vi "Keithley 6514 Digital Output Controls.vi"(0 "Resource In":refnum<visa-resource-name>, 1 "Check For SCPI Errors? (T)":bool=TRUE, 5 "Digital Output Control (Set Output Pattern:0)":u16(ring) items=["Set Output Pattern", "Clear Port Immediately", "Enable Auto-Clear Port", "Disable Auto-Clear Port", "Set Line-4 Mode Configuration"], 7 "4-Bit Digital\nOutput Pattern (1111b)":i8=15 min=0 max=15 step=1 format="%04b", 9 "Delay Pulse-Width for \nPass/Fail Pattern (0.0001 secs)":sgl=0.0001 min=0 max=60 step=0.0001 format="%.4f", 11 "error in (no error)":T1, 13 "Line 4 Mode (End of Test:T)":bool=TRUE, 14 "TTL Level for Busy (0:F)":bool) -> (4 "Resource Out":refnum<visa-resource-name>, 15 "error out":T1)   [LabVIEW 2009, in "Keithley 6514 LV 2009.lvlib"]
doc: "This VI is used to control the 4 digital output lines of the instrument. \n\nDigital Output Control:\n0 = Set Output Pattern\n1 = Clear Port Immediately\n2 = Enable Auto-Clear Port\n3 = Disable Auto-Clear Port\n4 = Set Line 4 Mode Configuration\n\n4-Bit Digital Output Pattern:\n0 to 15\n\nDelay Pulse-Width for Pass/Fail Pattern:\n0 to 60 (0.0001 Resolution)\n\nLine 4 Mode:\nTRUE = End of Test (EOT)'\nFALSE = Busy\n\nTTL Level for Busy:\nTRUE = 1 (HI)\nFALSE = 0 (LO)"
uses:
  Keithley 6514 LV 2009.lvlib
panel:
  # "End of Test\nBusy"
  # "1\n0"
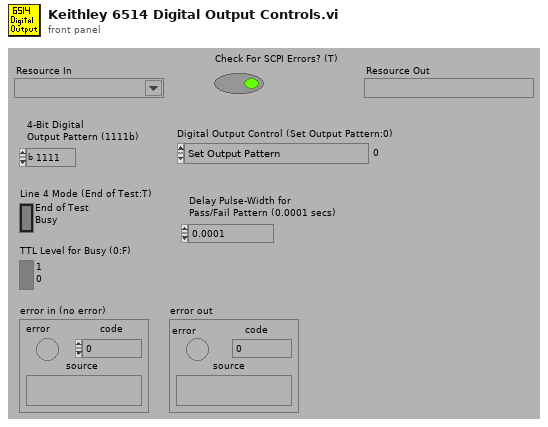
[diagram p1: front panel]
types:
  T1 = cluster{"error":bool, "code":i32, "source":string}
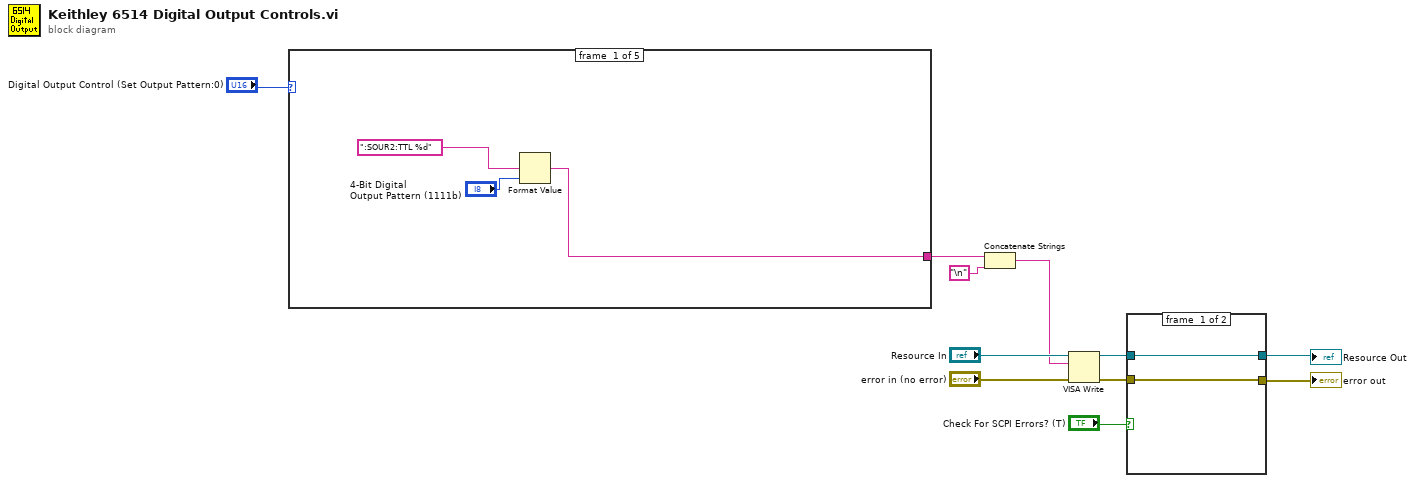
[diagram p0: block diagram]
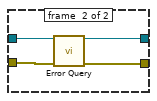
[diagram p2: hidden frame]
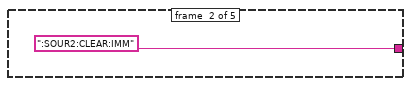
[diagram p3: hidden frame]
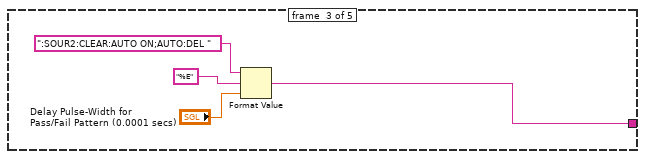
[diagram p4: hidden frame]
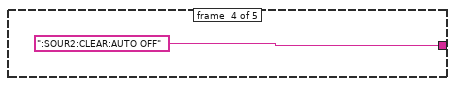
[diagram p5: hidden frame]
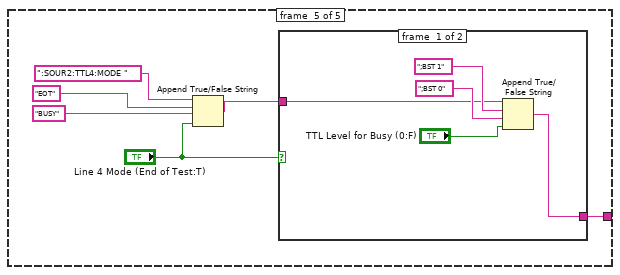
[diagram p6: hidden frame]
diagram:
  n1 = case shown="4" "Digital Output Control (Set Output Pattern:0)" {
    tunnel: [w12 ":SOUR2:CLEAR:IMM" w16 ":SOUR2:CLEAR:AUTO OFF" w21] -> w2
    frame #0 {
      n2 = Format Value(format string=":SOUR2:TTL %d", value (0)="4-Bit Digital\nOutput Pattern (1111b)") -> (output string=w12:string)  [unwired: 1 in]
    }
    frame #1 {
    }
    frame #2 {
      n3 = Format Value(string ("")=":SOUR2:CLEAR:AUTO ON;AUTO:DEL ", format string="%E", value (0)="Delay Pulse-Width for \nPass/Fail Pattern (0.0001 secs)") -> (output string=w16:string)
    }
    frame #3 {
    }
    frame #4 {
      n4 = Append True/False String(1:"Line 4 Mode (End of Test:T)", 2:"BUSY", 3:"EOT", 4:":SOUR2:TTL4:MODE ") -> (0:w22:string)
      n5 = case shown="True" "Line 4 Mode (End of Test:T)" {
        tunnel: [w28 w32] -> w21
        tunnel: w22 -> [w29 w32]
        frame #0 {
          n6 = Append True/False String(1:"TTL Level for Busy (0:F)", 2:";BST 0", 3:";BST 1", 4:w29) -> (0:w28:string)
        }
        frame #1 {
        }
      }
    }
  }
  n7 = Concatenate Strings(w2, "\n") -> (w1:string)
  n8 = VISA Write(VISA resource name="Resource In", write buffer=w1, error in (no error)="error in (no error)") -> (VISA resource name out=w7:refnum<visa-resource-name>, error out=w6:errorcluster)  [unwired: 1 out]
  n9 = case shown="False" "Check For SCPI Errors? (T)" {
    tunnel: w7 -> [w34 w38]
    tunnel: w6 -> [w33 w37]
    tunnel: [w34 w36] -> w5
    tunnel: [w33 w35] -> w4
    frame #0 {
    }
    frame #1 {
      n10 = call "Error Query.vi"("VISA Resource In"=w38, "error in (no error)"=w37) -> ("VISA Resource Out (dupl)"=w36:refnum<visa-resource-name>, "error out"=w35:errorcluster)  [unwired: 10 in, 2 out]
    }
  }
  "error out" <- w4
  "Resource Out" <- w5
